vi "Move.vi"(6 "Relative?":bool, 8 "error in (no error)":errorcluster, 9 "SetPosition":dbl, 10 "AxisNumber":u8, 11 "CS++Motor in":refnum<class "CS++Motor.lvclass">) -> (0 "error out":errorcluster, 3 "CS++Motor out":refnum<class "CS++Motor.lvclass">)   [LabVIEW 2016, in "CS++Motor.lvlib" / "CS++Motor.lvclass"]
doc: "Starts an absolute or relative movement of an axis."
uses:
  CS++Motor.lvclass
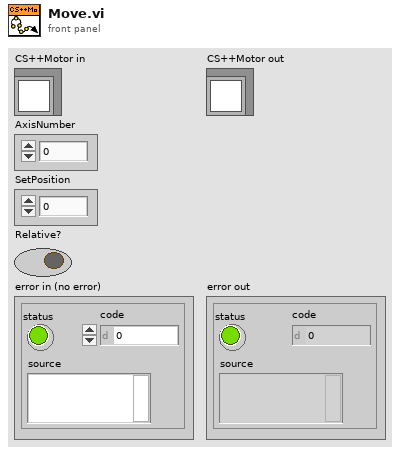
[diagram p1: front panel]
types:
  T1 = enum16{"NormalMovement", "ReferenceMovement", "StopMovement"}
  T2 = cluster{"MovementType":enum16{"NormalMovement", "ReferenceMovement", "StopMovement"}, "SetPosition":dbl, "Relative?":bool}
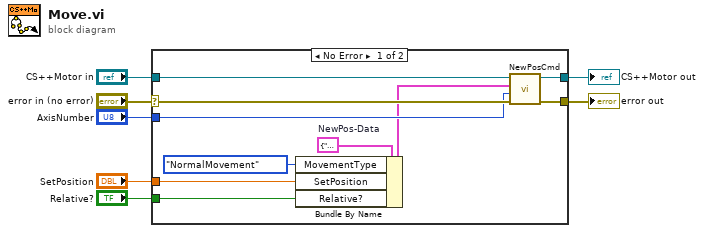
[diagram p0: block diagram]
diagram:
  n1 = case shown="No Error" "error in (no error)" {
    selector: "error in (no error)" -> [w13 w19]
    tunnel: [w12 w19] -> w6
    tunnel: [w11 w18] -> w4
    tunnel: "CS++Motor in" -> [w10 w18]
    tunnel: "AxisNumber" -> [w9 _]
    tunnel: "SetPosition" -> [w16 _]
    tunnel: "Relative?" -> [w15 _]
    frame No Error {
      w17 = T2 {"MovementType"=enum."NormalMovement", "SetPosition"=0.0, "Relative?"=FALSE}  # NewPos-Data
      n2 = Bundle By Name(cluster=w17, "MovementType"=T1."NormalMovement", "SetPosition"=w16, "Relative?"=w15) -> (w8:T2)
      n3 = call "NewPosCmd.vi"("error in (no error)"=w13, "AxisNumber"=w9, "NewPos-Data"=w8, "CS++Motor in"=w10) -> ("error out"=w12:errorcluster, "CS++Motor out"=w11:refnum<class "CS++Motor.lvclass">)  [unwired: 6 in]
    }
    frame Error {
    }
  }
  "error out" <- w6
  "CS++Motor out" <- w4
